vi "Write menu object array values.vi"(11 "Values":u16[](array[ring]) items=["Select one"]) -> (3 "Menu object array":T1 {"Object name" items=["Select one"]})   [LabVIEW 2019]
uses:
  Menu object array.ctl
  Menu object.ctl
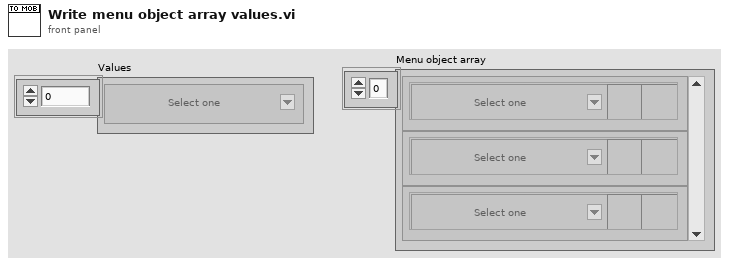
[diagram p1: front panel]
types:
  T1 = typedef "Menu object array.ctl" = T2[]
  T2 = typedef "Menu object.ctl" = cluster{"Object name":u16, "Open parameters":bool, "Remove Button":bool}
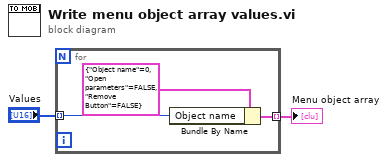
[diagram p0: block diagram]
diagram:
  n1 = for {
    tunnel: "Values" -> [w4] mode=indexing
    tunnel: [w3] -> w1 mode=indexing
    n2 = Bundle By Name(cluster=T2 {"Object name"=0, "Open parameters"=FALSE, "Remove Button"=FALSE} ("Menu object"), "Object name"=w4) -> (w3:T2)
  }
  "Menu object array" <- w1
